vi "Set Analog Replay Settings.vi"(8 "error in (no error)":errorcluster, 9 "Analog Replay Data Options":T1={"Input file"=path "", "Group"="", "Channel"="", "Reverse"=FALSE, "FPGA Memory Size"=enum."16,384", "Position reference"=enum."Crank angle", "Data selection method"=enum."Manual", "Offset"=0, "Samples"=0, "Missing teeth location"=0.0, "DataPlugin"=""}, 10 "Analog Replay Settings":T5={"Name"="", "DAC bipolar range (V)"=0.0, "Voltage below min speed"=0.0, "Min speed (RPM)"=0.0, "Voltage at min speed"=0.0, "Max speed (RPM)"=0.0, "Voltage at max speed"=0.0, "Negate playback voltage values at negative engine speed"=TRUE, "Allow run-time override of voltage scaling"=FALSE}, 11 "Analog Replay in":refnum<k24>) -> (0 "error out":errorcluster, 3 "Analog Replay out":refnum<k24>)   [LabVIEW 2015, in "Engine Simulation Toolkit SysDef API.lvlib"]
uses:
  Engine Simulation Toolkit SysDef API.lvlib
  Analog Replay Settings.ctl
  Analog Replay Data Options.ctl
  System Explorer/FPGA Mem Size.ctl
  System Explorer/Position Reference.ctl
  System Explorer/Data Replay Data Selection Method.ctl
  NationalInstruments.VeriStand.SystemDefinitionAPI
  System Explorer/File Load Dialog.ctl
  <vilib>/Platform/storage/utility/usiPluginInformation.ctl
  <vilib>/NI Veristand/Custom Device API/Custom Device Channel Type.ctl
  Shared/Constants and GUIDs.vi
  Shared/Properties.vi
  <vilib>/NI/NI VeriStand Advanced SysDef API/_SubVIs/SysDef.Property.Set.String.vi
  <vilib>/NI/NI VeriStand Advanced SysDef API/_SubVIs/SysDef.Property.Set.DBL.vi
  <vilib>/NI/NI VeriStand Advanced SysDef API/_SubVIs/SysDef.Property.Set.Boolean.vi
  Shared/Engine Simulation Toolkit Shared.lvlib
  System Explorer/Engine Simulation Toolkit System Explorer.lvlib
  <vilib>/NI Veristand/Custom Device API/Custom Device API.lvlib
  <vilib>/NI/NI VeriStand Advanced SysDef API/SysDef API/Advanced System Definition.lvlib
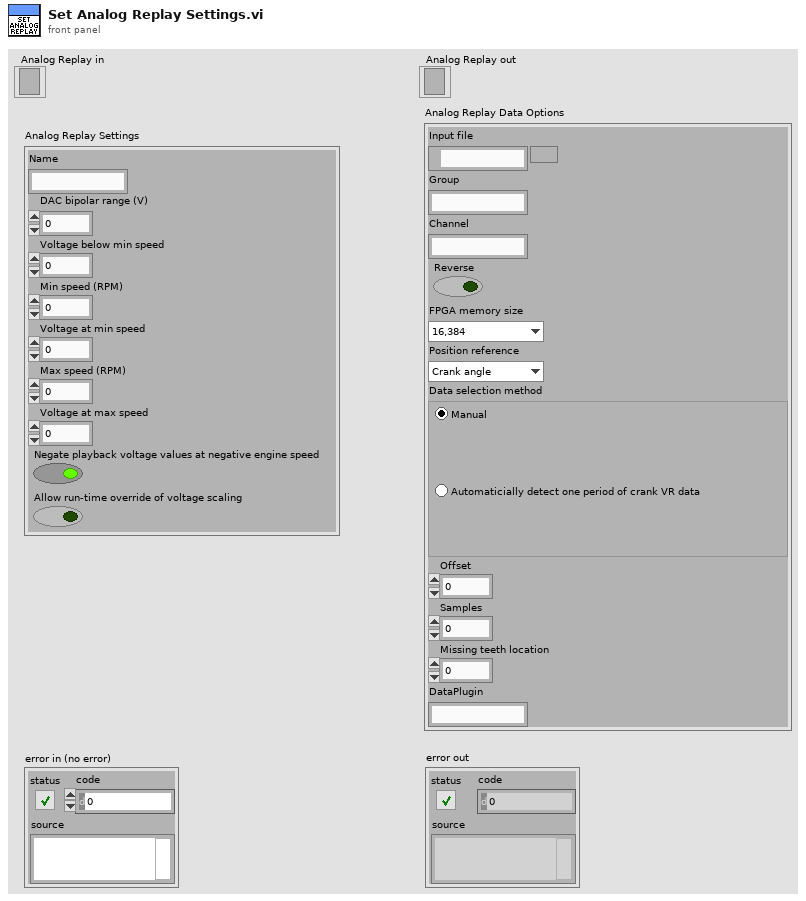
[diagram p1: front panel]
types:
  T1 = typedef "Engine Simulation Toolkit SysDef API.lvlib/Analog Replay Data Options.ctl" = cluster{"Input file":path, "Group":string, "Channel":string, "Reverse":bool, "FPGA Memory Size":T2, "Position reference":T3, "Data selection method":T4, "Offset":i32, "Samples":i32, "Missing teeth location":dbl, "DataPlugin":string}
  T2 = typedef "Engine Simulation Toolkit System Explorer.lvlib/FPGA Mem Size.ctl" = enum16{"65,536", "32,768", "16,384", "8,192", "4,096", "2,048", "1,024"}
  T3 = typedef "Engine Simulation Toolkit System Explorer.lvlib/Position Reference.ctl" = enum16{"Crank angle", "Cycle angle"}
  T4 = typedef "Engine Simulation Toolkit System Explorer.lvlib/Data Replay Data Selection Method.ctl" = enum32{"Manual", "AutoVRCrank"}
  T5 = typedef "Engine Simulation Toolkit SysDef API.lvlib/Analog Replay Settings.ctl" = cluster{"Name":string, "DAC bipolar range (V)":dbl, "Voltage below min speed":dbl, "Min speed (RPM)":dbl, "Voltage at min speed":dbl, "Max speed (RPM)":dbl, "Voltage at max speed":dbl, "Negate playback voltage values at negative engine speed":bool, "Allow run-time override of voltage scaling":bool}
  T6 = typedef "Engine Simulation Toolkit System Explorer.lvlib/File Load Dialog.ctl" = cluster{"File":path, "Group":string, "Channel":string, "DataPlugin":string, "MissingTeeth":dbl, "ErrState":string, "File Selected":bool, "Data Selection Method":T4, "Offset":i32, "Length":i32, "DataPlugins Info":T7[], "Controls":refnum<vi>[], "File Ref":refnum<k20>, "Groups":string[], "Channels":string[], "Groups Refs":refnum<k20>[], "Channel Refs":refnum<k20>[], "Cancelled":bool, "Position reference":T3, "FPGA memory size":T2, "GroupRef":refnum<k20>, "ChanRef":refnum<k20>, "Data":dbl[], "ReverseData":bool, "DispTwoRotations":bool, "cycle range":u16}
  T7 = typedef "usiPluginInformation.ctl" = cluster{"name":string, "version":string, "type":string, "read-only?":bool, "extensions":string[]}
  T8 = typedef "Custom Device API.lvlib/Custom Device Channel Type.ctl" = enum16{"Input", "Output"}
  T9 = typedef "Engine Simulation Toolkit Shared.lvlib/Channel.ctl" = cluster{"Name":string, "Units":string, "Default":dbl, "Description":string, "Scalable":bool}
  T10 = typedef "Custom Device API.lvlib/Custom Device Item Ref.ctl" = u64
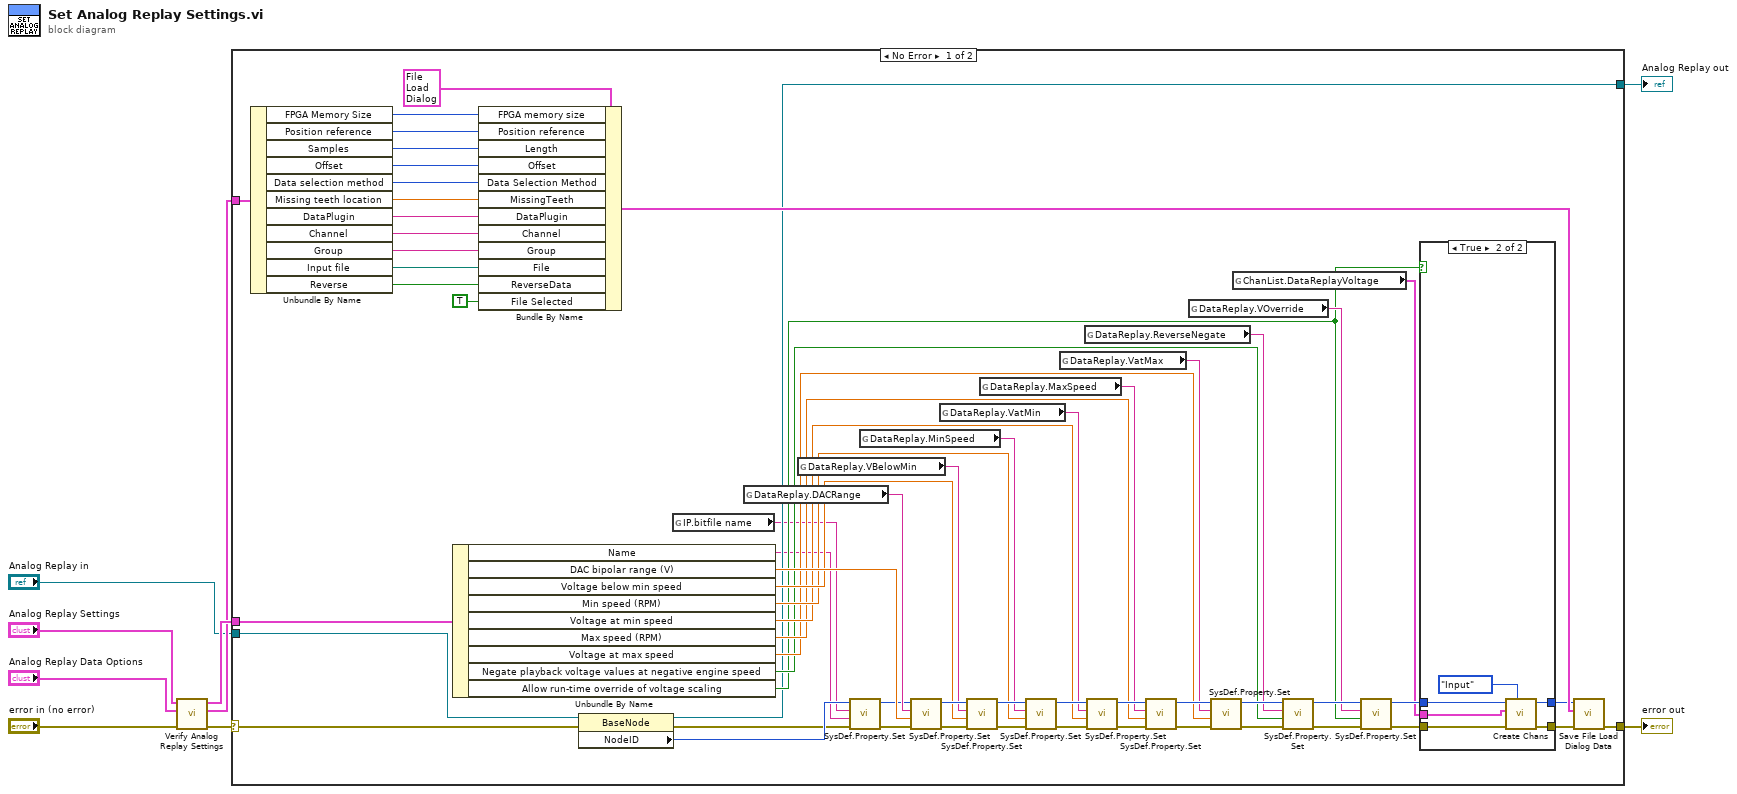
[diagram p0: block diagram]
diagram:
  n1 = call "Verify Analog Replay Settings.vi"("error in (no error)"="error in (no error)", "Analog Replay Data Options in"="Analog Replay Data Options", "Analog Replay Settings in"="Analog Replay Settings") -> ("error out"=w7:errorcluster, "Analog Replay Data Options out"=w3:T1, "Analog Replay Settings out"=w5:T5)  [unwired: 6 in]
  n2 = case shown="No Error" w7 {
    selector: w7 -> [w18 w80]
    tunnel: "Analog Replay in" -> [w17 w79]
    tunnel: [w16 w79] -> w1
    tunnel: [w19 w80] -> w9
    tunnel: w5 -> [w21 _]
    tunnel: w3 -> [w20 _]
    frame No Error {
      n3 = Unbundle By Name(w20) -> ("FPGA Memory Size"=w63:T2, "Position reference"=w64:T3, "Samples"=w23:i32, "Offset"=w24:i32, "Data selection method"=w26:T4, "Missing teeth location"=w25:dbl, "DataPlugin"=w22:string, "Channel"=w65:string, "Group"=w66:string, "Input file"=w67:path, "Reverse"=w68:bool)
      n4 = Unbundle By Name(w21) -> ("Name"=w12:string, "DAC bipolar range (V)"=w60:dbl, "Voltage below min speed"=w57:dbl, "Min speed (RPM)"=w49:dbl, "Voltage at min speed"=w47:dbl, "Max speed (RPM)"=w46:dbl, "Voltage at max speed"=w43:dbl, "Negate playback voltage values at negative engine speed"=w34:bool, "Allow run-time override of voltage scaling"=w32:bool)
      n5 = Bundle By Name(cluster=T6 {"File"=path "", "Group"="", "Channel"="", "DataPlugin"="", "MissingTeeth"=0.0, "ErrState"="", "File Selected"=FALSE, "Data Selection Method"=enum."Manual", "Offset"=0, "Length"=0, "DataPlugins Info"=[], "Controls"=[], "File Ref"=refnum, "Groups"=[], "Channels"=[], "Groups Refs"=[], "Channel Refs"=[], "Cancelled"=FALSE, "Position reference"=enum."Crank angle", "FPGA memory size"=enum."32,768", "GroupRef"=refnum, "ChanRef"=refnum, "Data"=[], "ReverseData"=FALSE, "DispTwoRotations"=FALSE, "cycle range"=720} ("FileDialog"), "FPGA memory size"=w63, "Position reference"=w64, "Length"=w23, "Offset"=w24, "Data Selection Method"=w26, "MissingTeeth"=w25, "DataPlugin"=w22, "Channel"=w65, "Group"=w66, "File"=w67, "ReverseData"=w68, "File Selected"=TRUE) -> (w69:T6)
      n6 = property class="BaseNode"(reference=w17, error in=w18) -> (reference out=w16:refnum<k24>, error out=w11:errorcluster, "NodeID"=w14:u64)
      n7 = global read "Properties.vi" "IP.bitfile name"() -> (w13:string)
      n8 = global read "Properties.vi" "DataReplay.DACRange"() -> (w61:string)
      n9 = global read "Properties.vi" "DataReplay.VBelowMin"() -> (w56:string)
      n10 = call-poly <vilib>:"SysDef.Property.Set.vi"("error in (no error)"=w11, "Value"=w12, "Property Name"=w13, "nodeID"=w14) -> ("error out"=w10:errorcluster, "nodeID out"=w15:u64)  [unwired: 6 in]
      n11 = global read "Properties.vi" "DataReplay.MinSpeed"() -> (w48:string)
      n12 = call-poly <vilib>:"SysDef.Property.Set.vi"("error in (no error)"=w10, "Value"=w60, "Property Name"=w61, "nodeID"=w15) -> ("error out"=w58:errorcluster, "nodeID out"=w59:u64)  [unwired: 6 in]
      n13 = global read "Properties.vi" "DataReplay.VatMin"() -> (w42:string)
      n14 = call-poly <vilib>:"SysDef.Property.Set.vi"("error in (no error)"=w58, "Value"=w57, "Property Name"=w56, "nodeID"=w59) -> ("error out"=w50:errorcluster, "nodeID out"=w51:u64)  [unwired: 6 in]
      n15 = global read "Properties.vi" "DataReplay.MaxSpeed"() -> (w41:string)
      n16 = call-poly <vilib>:"SysDef.Property.Set.vi"("error in (no error)"=w50, "Value"=w49, "Property Name"=w48, "nodeID"=w51) -> ("error out"=w55:errorcluster, "nodeID out"=w54:u64)  [unwired: 6 in]
      n17 = global read "Properties.vi" "DataReplay.VatMax"() -> (w40:string)
      n18 = global read "Properties.vi" "DataReplay.ReverseNegate"() -> (w35:string)
      n19 = call-poly <vilib>:"SysDef.Property.Set.vi"("error in (no error)"=w55, "Value"=w47, "Property Name"=w42, "nodeID"=w54) -> ("error out"=w53:errorcluster, "nodeID out"=w52:u64)  [unwired: 6 in]
      n20 = call-poly <vilib>:"SysDef.Property.Set.vi"("error in (no error)"=w53, "Value"=w46, "Property Name"=w41, "nodeID"=w52) -> ("error out"=w45:errorcluster, "nodeID out"=w44:u64)  [unwired: 6 in]
      n21 = global read "Properties.vi" "DataReplay.VOverride"() -> (w33:string)
      n22 = call-poly <vilib>:"SysDef.Property.Set.vi"("error in (no error)"=w45, "Value"=w43, "Property Name"=w40, "nodeID"=w44) -> ("error out"=w39:errorcluster, "nodeID out"=w38:u64)  [unwired: 6 in]
      n23 = global read "Constants and GUIDs.vi" "ChanList.DataReplayVoltage"() -> (w27:T9[])
      n24 = call-poly <vilib>:"SysDef.Property.Set.vi"("error in (no error)"=w39, "Value"=w34, "Property Name"=w35, "nodeID"=w38) -> ("error out"=w37:errorcluster, "nodeID out"=w36:u64)  [unwired: 6 in]
      n25 = call-poly <vilib>:"SysDef.Property.Set.vi"("error in (no error)"=w37, "Value"=w32, "Property Name"=w33, "nodeID"=w36) -> ("error out"=w31:errorcluster, "nodeID out"=w30:u64)  [unwired: 6 in]
      n26 = case shown="True" w32 {
        tunnel: w31 -> [w72 w76]
        tunnel: w30 -> [w71 w77]
        tunnel: [w72 w75] -> w29
        tunnel: [w71 w74] -> w28
        tunnel: w27 -> [_ w73]
        frame False {
        }
        frame True {
          n27 = call "Create Chans.vi"("Type"=Custom_Device_Channel_Type."Input", "error in (no error)"=w76, "Channels"=w73, "Section Ptr"=w77) -> ("error out"=w75:errorcluster, "Section Ptr dup"=w74:T10)  [unwired: 4 in, 2 out]
        }
      }
      n28 = call "Save File Load Dialog Data.vi"("error in (no error)"=w29, "FileDialog"=w69, "Node Ptr"=w28) -> ("error out"=w19:errorcluster)  [unwired: 8 in]
    }
    frame Error {
    }
  }
  "error out" <- w9
  "Analog Replay out" <- w1
